vi "Aquitaine Editor.vi"(10 "Project Info":T5, 11 "Path":path) -> ()   [LabVIEW 2025]
uses:
  Types/Decision Tree.ctl
  Types/Sequencing Tree Node.ctl
  Types/Single Cmd Info.ctl
  <vilib>/picture/picture.llb/imagedata.ctl
  <vilib>/Utility/miscctls.llb/LVPositionTypeDef.ctl
panel:
  in  "Test Tree":T1
  out "AQT PATH NAME":string
  in  "Refresh":bool
  in  "Export to Draw Menu":bool
  in  "Close":bool
  out "Tree":picture
  out "Sequencing Command Palette":picture
  in  "Save":bool
  in  "Path References":i32[](listbox)
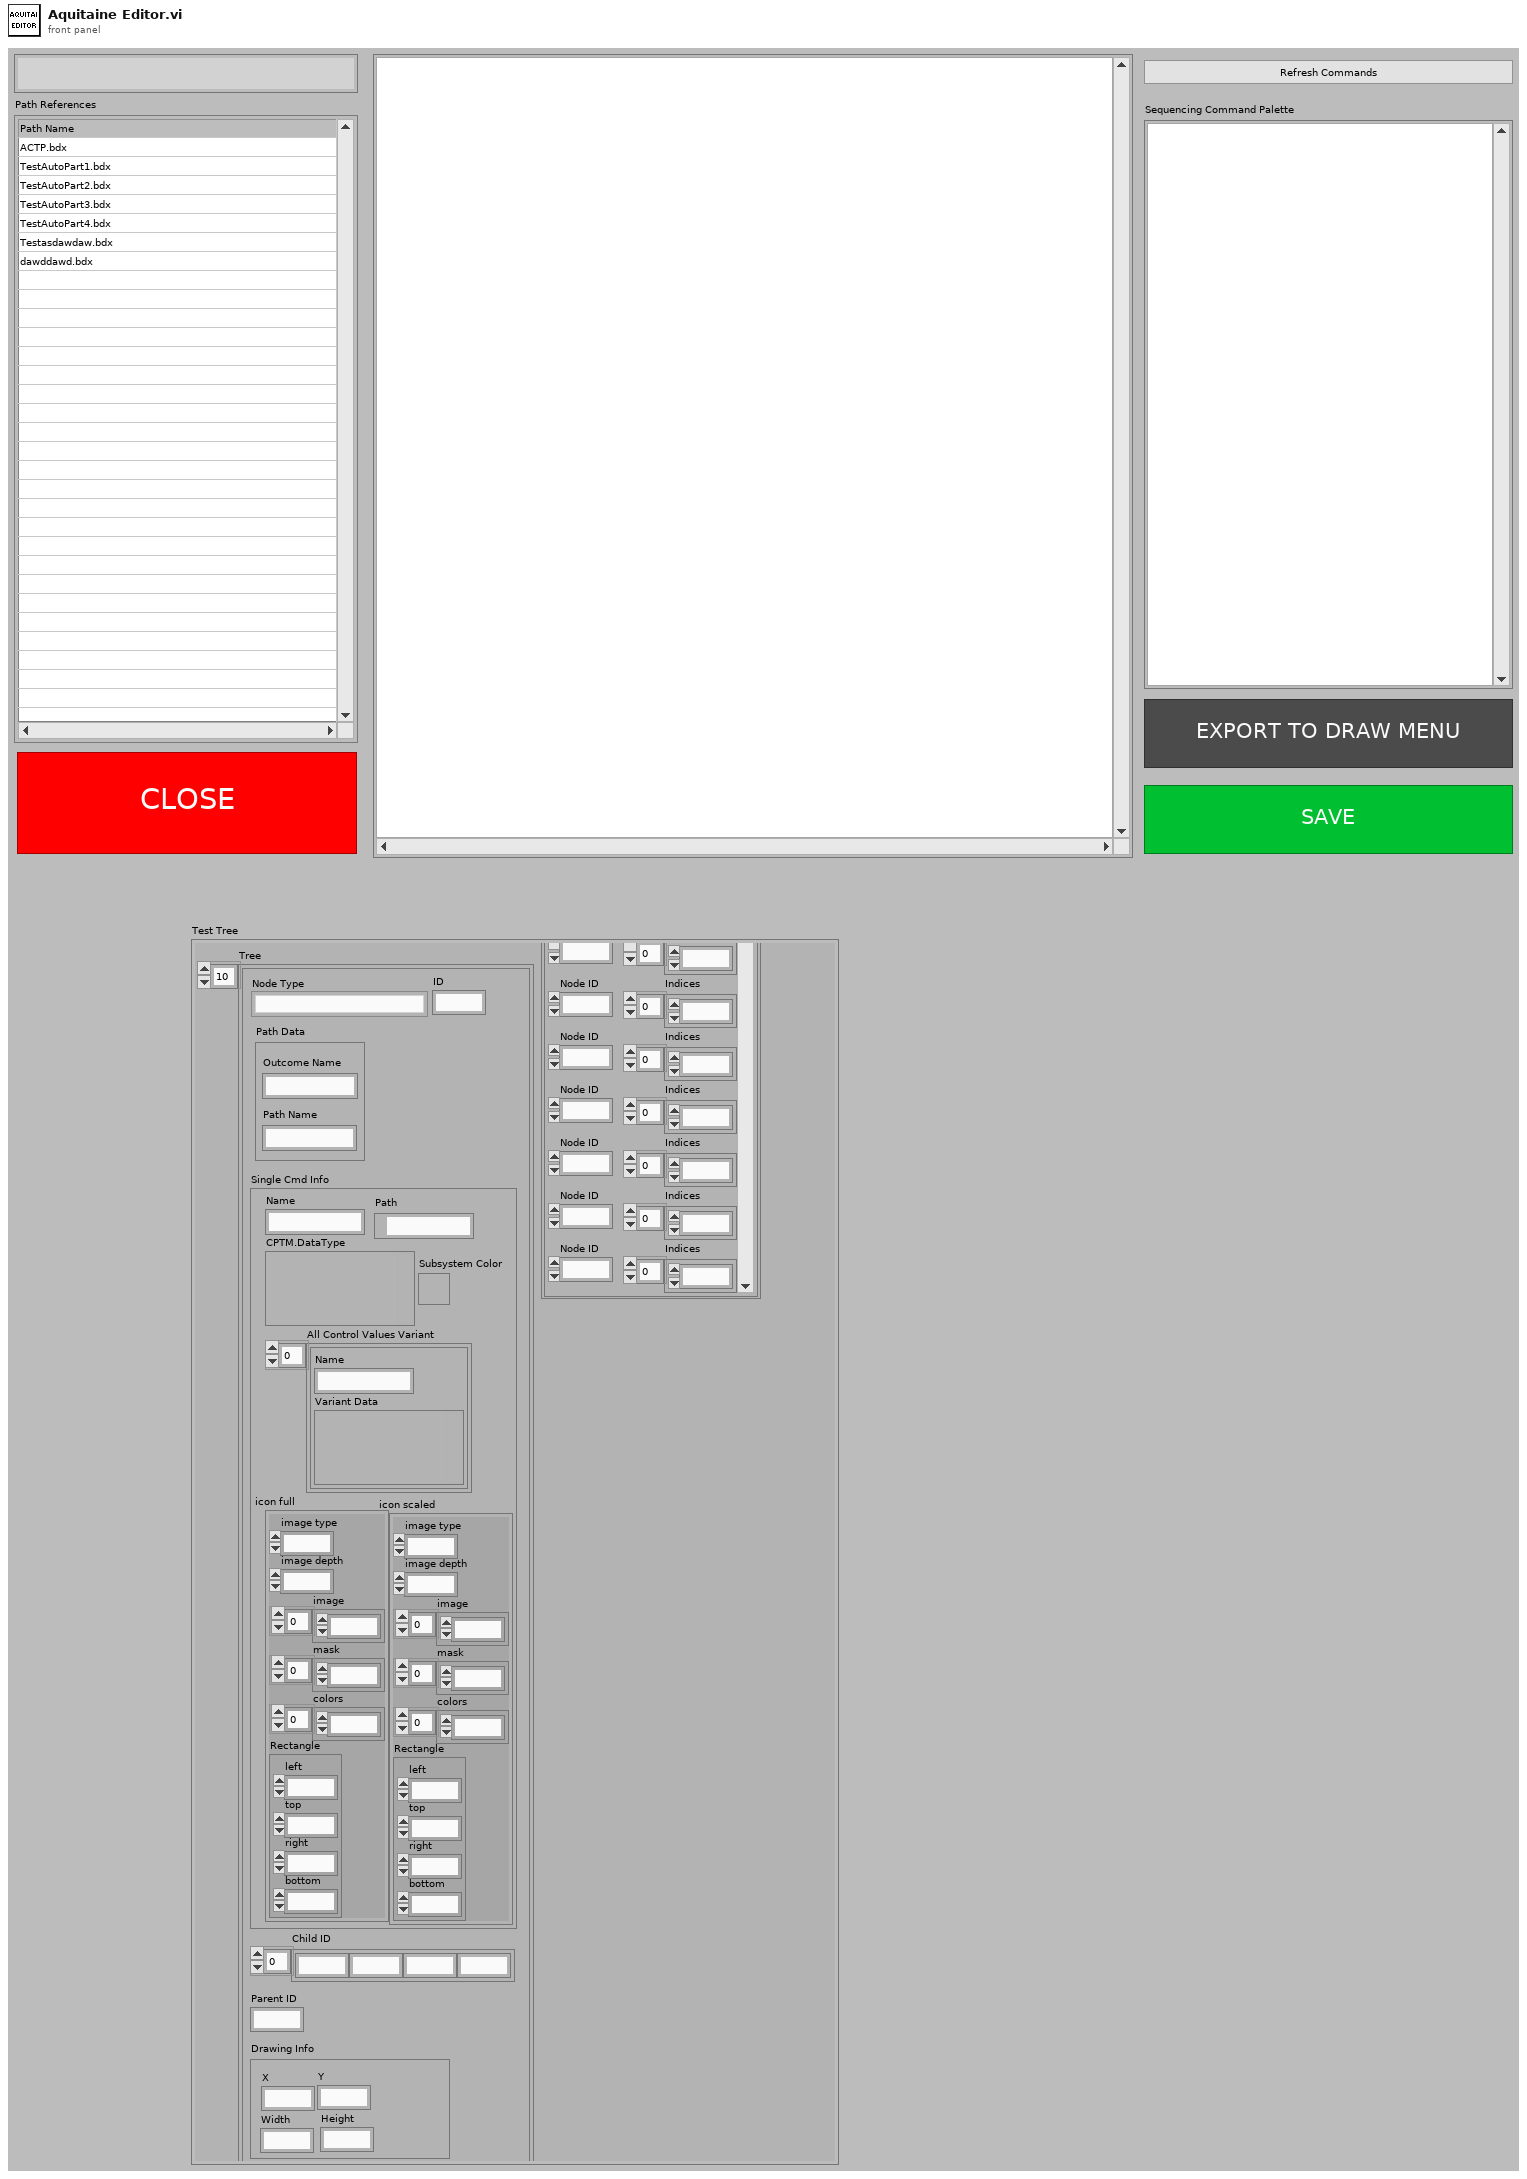
[diagram p1: front panel]
types:
  T1 = typedef "Decision Tree.ctl" = cluster{"Tree":T2[], "Node To Index Lookup Map":map{i16, i16[]}}
  T2 = typedef "Sequencing Tree Node.ctl" = cluster{"Node Type":enum16{"Path", "Command", "Leaf"}, "ID":i16, "Path Data":cluster{"Path Name":string, "Outcome Name":string}, "Single Cmd Info":T3, "Child ID":i32[], "Parent ID":i32, "Drawing Info":cluster{"X":i32, "Y":i32, "Width":i32, "Height":i32}}
  T3 = typedef "Single Cmd Info.ctl" = cluster{"Name":string, "CPTM.DataType":variant, "All Control Values Variant":cluster{"Name":string, "Variant Data":variant}[], "icon full":T4, "icon scaled":T4, "Path":path, "Subsystem Color":u32}
  T4 = typedef "imagedata.ctl" = cluster{"image type":i32, "image depth":i32, "image":u8[], "mask":u8[], "colors":u32[], "Rectangle":cluster{"left":i16, "top":i16, "right":i16, "bottom":i16}}
  T5 = cluster{"Targets":refnum<vi>[], "Paths":path[], "Projects":u16}
  T6 = typedef "LVPositionTypeDef.ctl" = cluster{"Left":i32, "Top":i32}
  T7 = cluster{"Path References":path[], "Decision Tree":T1}
  T8 = typedef "LVBoundsTypeDef.ctl" = cluster{"Width":u32, "Height":u32}
  T9 = cluster{"Shift":bool, "Ctrl":bool, "Alt":bool, "Cmd":bool, "Opt":bool}
  T10 = typedef "LVMouseTypeDef.ctl" = cluster{"Mouse Position":cluster{"X":i32, "Y":i32}, "Mouse Modifiers":cluster{"Button Down":bool, "Shift Mod":bool, "Menu Mod":bool, "Option Mod":bool}}
  T11 = cluster{"Tree Out":T2[], "map out":map{i16, i16[]}}
  T12 = typedef "eventvkey.ctl" = enum16{"ASCII", "Enter", "Return", "Shift", "Ctrl", "Alt", "Cmd", "Opt", "Caps", "NumLock", "Clear", "Break", "Up", "Down", "Left", "Right", "Insert", "Delete", "Home", "End", "PageUp", "PageDown", "Escape", "Help", "Pause", "ScrollLock", "F1", "F2", "F3", "F4", "F5", "F6", "F7", "F8", "F9", "F10", "F11", "F12", "F13", "F14", "F15", "F16", "F17", "F18", "F19", "F20", "F21", "F22", "F23", "F24", "Play", "VolumeUp", "VolumeDown", "Mute", "Two Byte Char"}
  T13 = typedef "LVPoint32TypeDef.ctl" = cluster{"Horizontal":i32, "Vertical":i32}
  T14 = typedef "LVRowAndColumnTypeDef.ctl" = cluster{"Row":i32, "Column":i32}
  T15 = cluster{"Tree":T2[], "Node To Index Lookup Map":map{i16, i16[]}}
  T16 = cluster{"Name":string, "CPTM.DataType":variant, "Get All Control Values Variant":cluster{"Name":string, "Variant Data":variant}[], "Color 256":T4, "Subsystem Color":u32}[]
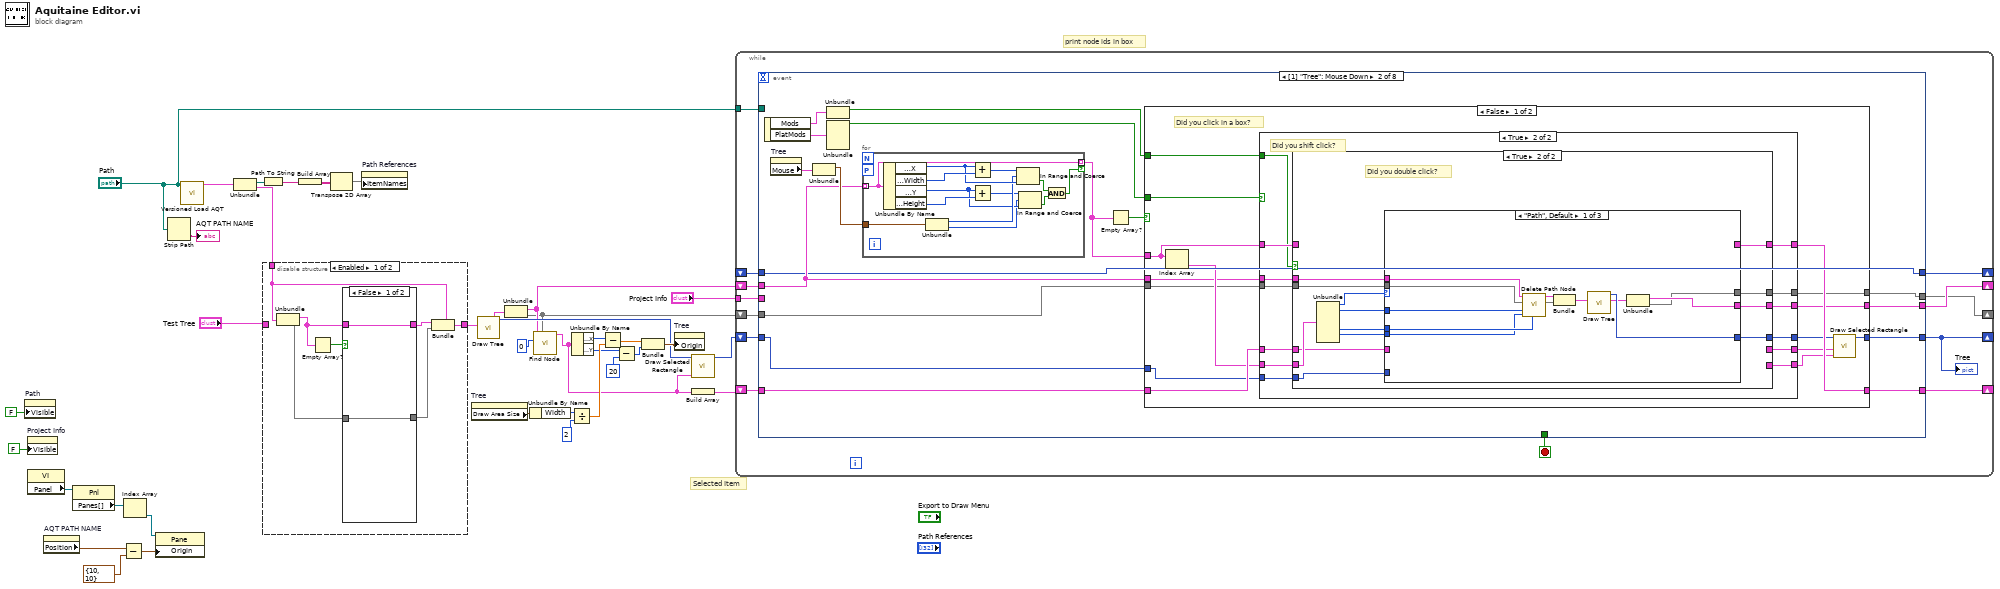
[diagram p0: block diagram]
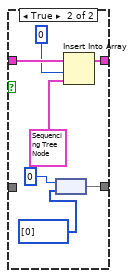
[diagram p2: hidden frame]
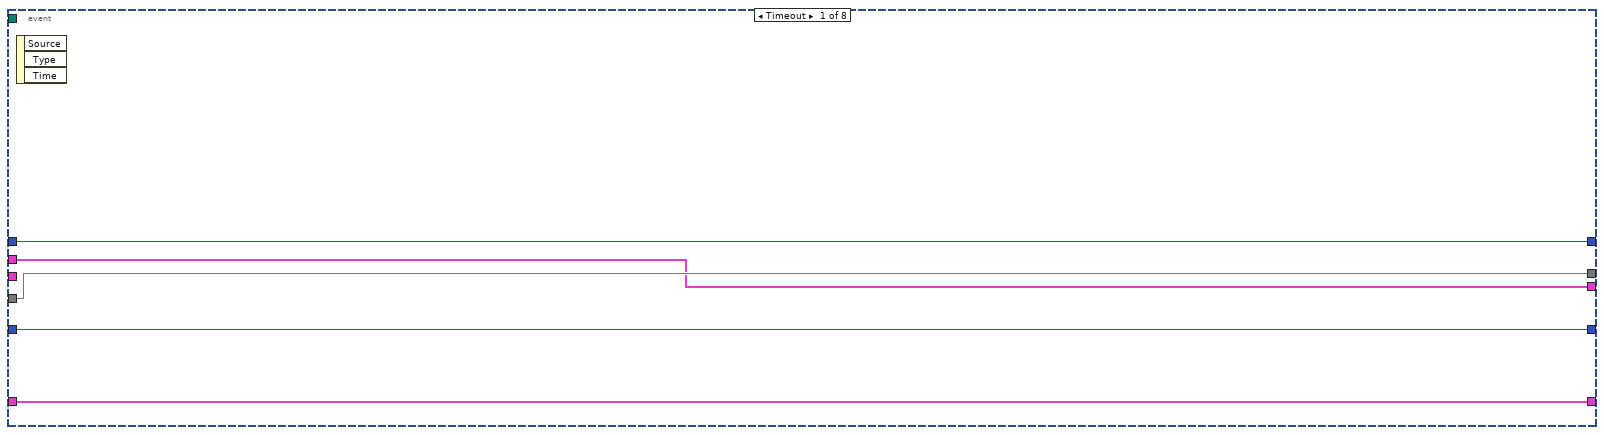
[diagram p4: hidden frame]
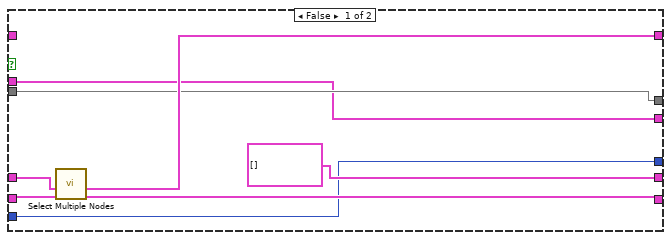
[diagram p6: hidden frame]
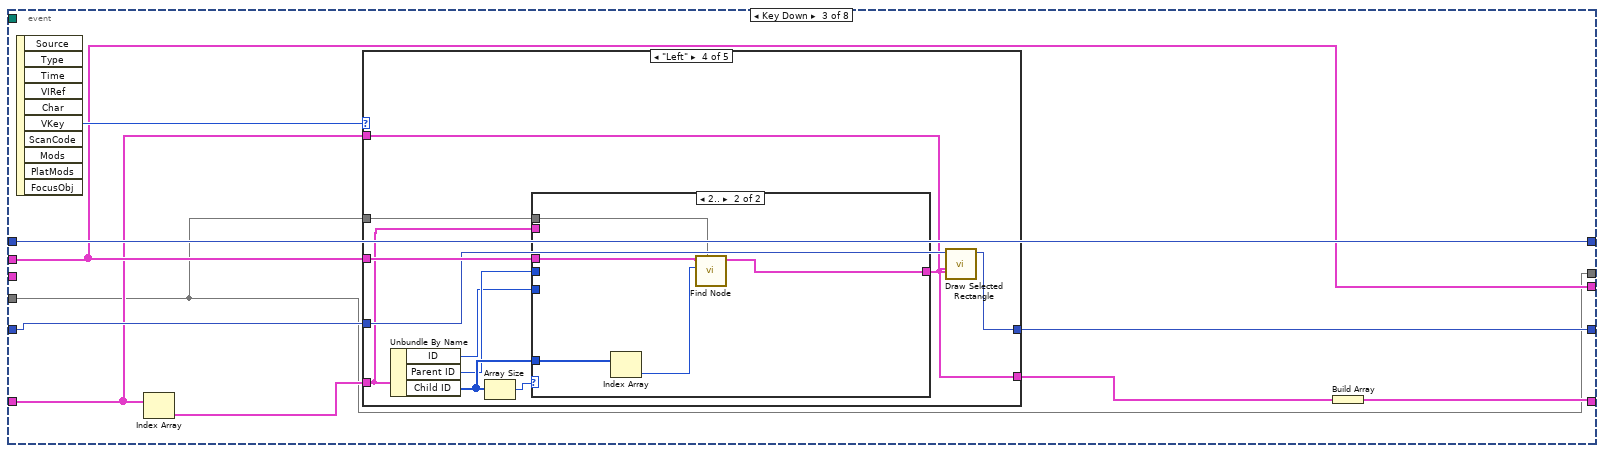
[diagram p10: hidden frame]
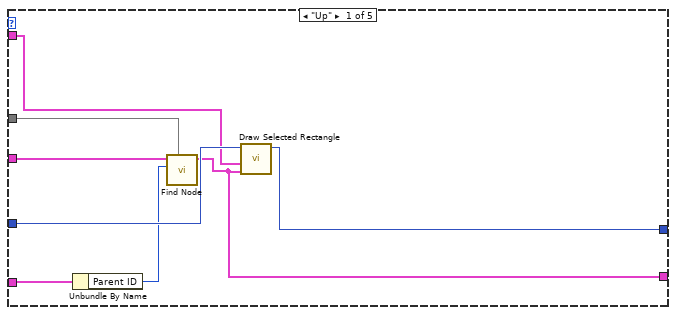
[diagram p11: hidden frame]
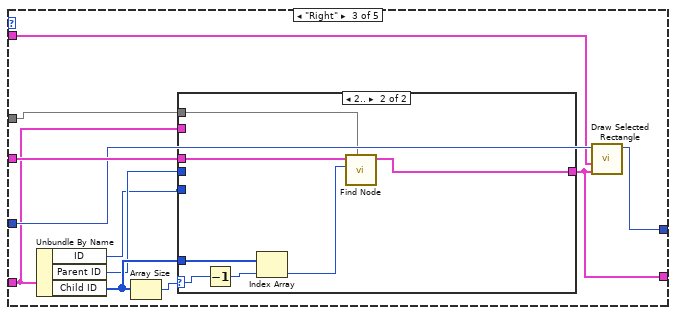
[diagram p13: hidden frame]
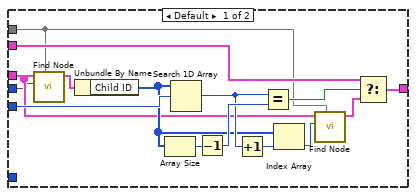
[diagram p14: hidden frame]
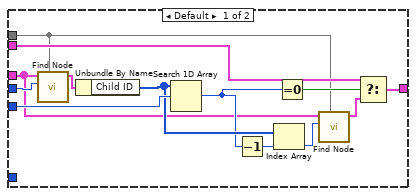
[diagram p15: hidden frame]
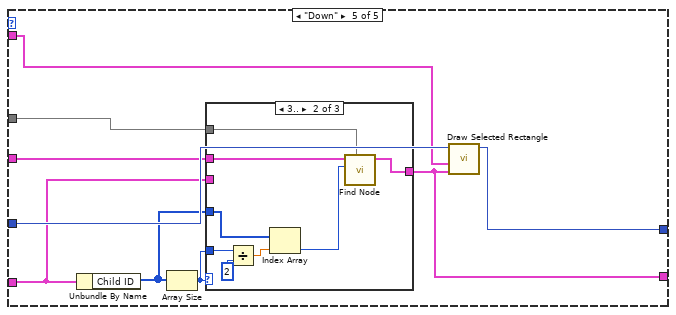
[diagram p16: hidden frame]
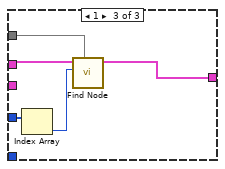
[diagram p18: hidden frame]
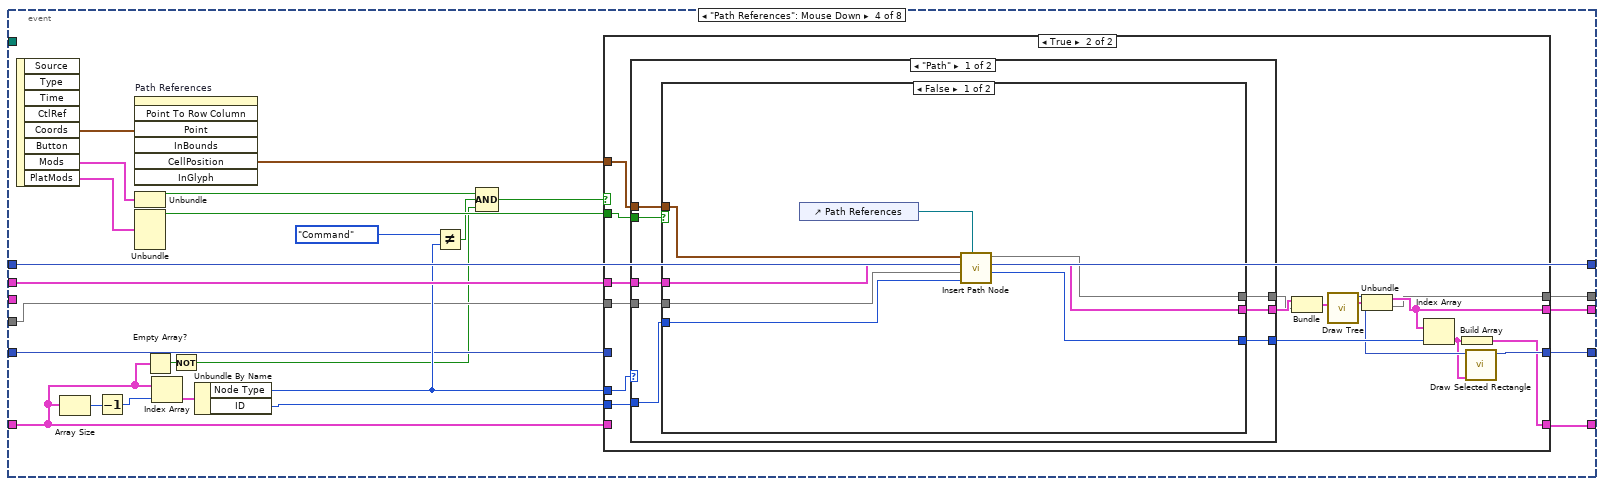
[diagram p19: hidden frame]
diagram:
  # "print node ids in box"
  # "Selected Item"
  n1 = property on="Path" class="Path"("Visible"=FALSE) -> ()  [unwired: 2 in, 2 out]
  n2 = property on="Project Info" class="Clust (strict)"("Visible"=FALSE) -> ()  [unwired: 2 in, 2 out]
  n3 = property class="VI"() -> ("Panel"=w27:refnum<vi>)  [unwired: 2 in, 2 out]
  n4 = property on="AQT PATH NAME" class="Str"() -> ("Position"=w23:T6)  [unwired: 2 in, 2 out]
  n5 = property class="Pnl"(reference=w27) -> ("Panes[]"=w26:refnum<vi>[])  [unwired: 1 in, 2 out]
  n6 = Subtract(x=w23, y=T6 {"Left"=10, "Top"=10}) -> (x-y=w22:T6)
  n7 = Index Array(array=w26) -> (element=w25:refnum<vi>)  [unwired: 1 in]
  n8 = property class="Pane"(reference=w25, "Origin"=w22) -> ()  [unwired: 1 in, 2 out]
  n9 = Strip Path(path="Path") -> (name=→"AQT PATH NAME":string)  [unwired: 1 out]
  n10 = call "Versioned Load AQT.vi"("Path"="Path") -> ("data"=w37:T7)  [unwired: 10 in]
  n11 = Unbundle(w37) -> ("Path References"=w36:path[], "Decision Tree"=w21:T1)
  n12 = Path To String(path=w36) -> (string=w35:string[])
  n13 = disable-structure shown="Enabled" {
    disable-tunnel: w21 -> [w41 _]
    disable-tunnel: [w40 w54] -> w8
    disable-tunnel: "Test Tree" -> [_ w54]
    frame Enabled {
      n14 = Unbundle(w41) -> ("Tree"=w43:T2[], "Node To Index Lookup Map"=w39:map{i16, i16[]})
      n15 = Empty Array?(array=w43) -> (empty?=w44:bool)
      n16 = case shown="False" w44 {
        tunnel: w43 -> [w46 w53]
        tunnel: [w46 w50] -> w42
        tunnel: w39 -> [w45 _]
        tunnel: [w45 w49] -> w38
        frame False {
        }
        frame True {
          n17 = node(i16 0, i16[] [0]) -> (w49:map{i16, i16[]})
          n18 = Insert Into Array(array=w53, index=0, new element=T2 {"Node Type"=enum."Leaf", "ID"=0, "Path Data"={"Path Name"="", "Outcome Name"=""}, "Single Cmd Info"={"Name"="", "CPTM.DataType"=variant, "All Control Values Variant"=[], "icon full"={"image type"=0, "image depth"=0, "image"=[], "mask"=[], "colors"=[], "Rectangle"={"left"=0, "top"=0, "right"=0, "bottom"=0}}, "icon scaled"={"image type"=0, "image depth"=0, "image"=[], "mask"=[], "colors"=[], "Rectangle"={"left"=0, "top"=0, "right"=0, "bottom"=0}}, "Path"=path "", "Subsystem Color"=16777216}, "Child ID"=[], "Parent ID"=0, "Drawing Info"={"X"=0, "Y"=0, "Width"=0, "Height"=0}} ("new element/subarray")) -> (w50:T2[])
        }
      }
      n19 = Bundle(cluster=w41, "Tree"=w42, "Node To Index Lookup Map"=w38) -> (w40:T1)
    }
    frame Disabled {
    }
  }
  n20 = Build Array(w35) -> (w34:string[][])
  n21 = Transpose 2D Array(2D array=w34) -> (transposed array=w33:string[][])
  n22 = property on="Path References" class="MCListbox (strict)"("ItemNames"=w33) -> ()  [unwired: 2 in, 2 out]
  n23 = property on="Tree" class="Pict"() -> ("Draw Area Size"=w17:T8)  [unwired: 2 in, 2 out]
  n24 = call "Draw Tree.vi"("Sequencing Data"=w8) -> ("Tree"=w5:T1, "2D Picture"=w10:picture)  [unwired: 9 in]
  n25 = Unbundle(w5) -> ("Tree"=w2:T2[], "Node To Index Lookup Map"=w1:map{i16, i16[]})
  n26 = Unbundle By Name(w17) -> ("Width"=w16:u32)
  n27 = call "Find Node.vi"("Node To Index Lookup Map"=w1, "ID"=0, "Tree"=w2) -> ("Node"=w3:T2)  [unwired: 7 in, 1 out]
  n28 = Divide(x=w16, y=u32 2) -> (x/y=w14:dbl)
  n29 = Unbundle By Name(w3) -> ("Drawing Info.X"=w19:i32, "Drawing Info.Y"=w12:i32)
  n30 = Subtract(x=w19, y=w14) -> (x-y=w18:dbl)
  n31 = Subtract(x=w12, y=20) -> (x-y=w13:i32)
  n32 = Bundle(w18, w13) -> (w20:cluster{dbl, i32})  [unwired: 1 in]
  n33 = property on="Tree" class="Pict"("Origin"=w20) -> ()  [unwired: 2 in, 2 out]
  n34 = call "Draw Selected Rectangle.vi"("New Node"=w3, "2D Picture"=w10) -> ("Decision Tree Out"=w9:picture)  [unwired: 9 in]
  n35 = Build Array(w3) -> (w6:T2[])
  n36 = while {
    tunnel: "Path" -> [w67]
    tunnel: "Project Info" -> [w65]
    shift-right: [w64] -> _
    shift-left: _ -> [w63]
    shift-right: [w58] -> _
    shift-left: w9 -> [w62]
    shift-right: [w59] -> _
    shift-left: w6 -> [w61]
    shift-right: [w56] -> _
    shift-left: w2 -> [w60]
    shift-right: [w55] -> _
    shift-left: w1 -> [w57]
    stop <- w66 stop-if-true
    n37 = event shown="[1] \"Tree\": Mouse Down" {
      selector: _ -> [_ _ _ _ _ _ _ _]
      dyn-events: _ -> [_ _ _ _ _ _ _ _]
      timeout: _ -> [_ _ _ _ _ _ _ _]
      tunnel: w67 -> [_ _ _ _ _ _ _ _]
      tunnel: [_ _ _ _ w392 _ _ w450] -> w66
      tunnel: w65 -> [_ _ _ _ _ w399 _ _]
      tunnel: [w72 w73 w190 w310 w391 w398 w427 w449] -> w64
      tunnel: w63 -> [w72 w73 w190 w310 w391 w397 w427 w449]
      tunnel: [w71 w80 w186 w290 w390 w396 w426 w448] -> w58
      tunnel: w62 -> [w71 w81 w188 w289 w390 w396 w426 w448]
      tunnel: w61 -> [w70 w84 w182 w288 w389 w395 w425 w447]
      tunnel: w60 -> [w68 w78 w187 w306 w387 w393 w423 w445]
      tunnel: [w70 w83 w183 w291 w389 w395 w425 w447] -> w59
      tunnel: w57 -> [w69 w77 w181 w294 w388 w394 w424 w446]
      tunnel: [w68 w75 w187 w293 w387 w393 w423 w445] -> w56
      tunnel: [w69 w74 w181 w292 w388 w394 w424 w446] -> w55
      event Timeout {
        n38 = event-data() -> ()  [unwired: 1 in, 3 out]
      }
      event "Tree": Mouse Down {
        n39 = event-data() -> ("Mods"=w88:cluster{"Double Click":bool, "Menu Key":bool}, "PlatMods"=w87:T9)  [unwired: 1 in]
        n40 = property on="Tree" class="Pict"() -> ("Mouse"=w89:T10)  [unwired: 2 in, 2 out]
        n41 = Unbundle(w89) -> ("Mouse Position"=w86:cluster{"X":i32, "Y":i32})  [unwired: 1 out]
        n42 = Unbundle(w88) -> ("Double Click"=w76:bool)  [unwired: 1 out]
        n43 = Unbundle(w87) -> ("Shift"=w79:bool)  [unwired: 4 out]
        n44 = for {
          workers-P: _ -> [_]
          tunnel: w78 -> [w91] mode=indexing
          tunnel: w86 -> [w102]
          tunnel: [w91] -> w82 mode=indexing if=w90
          n45 = Unbundle By Name(w91) -> ("Drawing Info.X"=w99:i32, "Drawing Info.Width"=w101:i32, "Drawing Info.Y"=w95:i32, "Drawing Info.Height"=w97:i32)
          n46 = Unbundle(w102) -> ("X"=w98:i32, "Y"=w94:i32)
          n47 = Add(x=w99, y=w101) -> (x+y=w100:i32)
          n48 = Add(x=w95, y=w97) -> (x+y=w96:i32)
          n49 = In Range and Coerce(upper limit=w100, x=w98, lower limit=w99) -> (In Range?=w92:bool)  [unwired: 1 out]
          n50 = In Range and Coerce(upper limit=w96, x=w94, lower limit=w95) -> (In Range?=w93:bool)  [unwired: 1 out]
          n51 = And(x=w92, y=w93) -> (x .and. y?=w90:bool)
        }
        n52 = Empty Array?(array=w82) -> (empty?=w85:bool)
        n53 = case shown="False" w85 {
          tunnel: w84 -> [w114 w180]
          tunnel: [w115 w180] -> w83
          tunnel: w82 -> [w116 _]
          tunnel: w81 -> [w104 w179]
          tunnel: [w117 w179] -> w80
          tunnel: w79 -> [w110 _]
          tunnel: w78 -> [w109 w177]
          tunnel: w77 -> [w108 w178]
          tunnel: w76 -> [w107 _]
          tunnel: [w106 w177] -> w75
          tunnel: [w105 w178] -> w74
          frame False {
            # "Did you click in a box?"
            n54 = Index Array(array=w116) -> (element=w112:T2)  [unwired: 1 in]
            n55 = case shown="True" w110 {
              tunnel: w116 -> [w123 w135]
              tunnel: [w123 w131] -> w115
              tunnel: w114 -> [w122 w132]
              tunnel: [w122 w136] -> w113
              tunnel: w112 -> [w121 w134]
              tunnel: [w121 w133] -> w111
              tunnel: w109 -> [w119 w130]
              tunnel: w108 -> [w120 w129]
              tunnel: w107 -> [_ w128]
              tunnel: [w119 w127] -> w106
              tunnel: [w120 w126] -> w105
              tunnel: w104 -> [w118 w125]
              tunnel: [w118 w124] -> w103
              frame False {
              }
              frame True {
                # "Did you shift click?"
                n56 = case shown="True" w128 {
                  tunnel: [T2[] [] ("Array") _] -> w136
                  tunnel: [w141 _] -> w133
                  tunnel: w135 -> [_ _]
                  tunnel: w134 -> [w142 w157]
                  tunnel: w132 -> [w143 w153]
                  tunnel: [w140 w152] -> w131
                  tunnel: w130 -> [w138 w155]
                  tunnel: w129 -> [w139 w154]
                  tunnel: [w138 w148] -> w127
                  tunnel: [w139 w147] -> w126
                  tunnel: w125 -> [w137 w146]
                  tunnel: [w137 w145] -> w124
                  frame False {
                    n57 = call "Select Multiple Nodes.vi"("Node to Select"=w142, "Selected Nodes"=w143) -> ("New Node"=w141:T2, "Selected Nodes New"=w140:T2[])  [unwired: 8 in]
                  }
                  frame True {
                    # "Did you double click?"
                    n58 = Unbundle(w157) -> ("Node Type"=w156:enum16{"Path", "Command", "Leaf"}, "ID"=w149:i16, "Child ID"=w150:i32[], "Parent ID"=w151:i32)  [unwired: 3 out]
                    n59 = case shown="\"Path\", Default" w156 {
                      tunnel: w155 -> [w168 w171 w175]
                      tunnel: w154 -> [w167 w172 w176]
                      tunnel: w153 -> [_ w173 _]
                      tunnel: [_ w173 _] -> w152
                      tunnel: w151 -> [w165 _ _]
                      tunnel: w150 -> [w169 _ _]
                      tunnel: w149 -> [w166 _ _]
                      tunnel: [w159 w171 w175] -> w148
                      tunnel: [w158 w172 w176] -> w147
                      tunnel: w146 -> [_ w170 w174]
                      tunnel: [w161 w170 w174] -> w145
                      frame "Path", Default {
                        n60 = call "Delete Path Node.vi"("Child ID"=w169, "Parent ID"=w165, "ID"=w166, "Node To Index Lookup Map"=w167, "Tree"=w168) -> ("map out"=w163:map{i16, i16[]}, "Tree Out"=w164:T2[])  [unwired: 5 in]
                        n61 = Bundle("Tree Out"=w164, "map out"=w163) -> (w162:T11)  [unwired: 1 in]
                        n62 = call "Draw Tree.vi"("Sequencing Data"=w162) -> ("Tree"=w160:T1, "2D Picture"=w161:picture)  [unwired: 9 in]
                        n63 = Unbundle(w160) -> ("Tree"=w159:T2[], "Node To Index Lookup Map"=w158:map{i16, i16[]})
                      }
                      frame "Leaf" {
                      }
                      frame "Command" {
                      }
                    }
                  }
                }
              }
            }
            n64 = call "Draw Selected Rectangle.vi"("New Node"=w111, "Prev. Node"=w113, "2D Picture"=w103) -> ("Decision Tree Out"=w117:picture)  [unwired: 8 in]
          }
          frame True {
          }
        }
      }
      event Key Down {
        n65 = event-data() -> ("VKey"=w189:T12)  [unwired: 1 in, 9 out]
        n66 = Index Array(array=w182) -> (element=w185:T2)  [unwired: 1 in]
        n67 = case shown="\"Left\"" w189 {
          tunnel: w188 -> [w198 w200 w208 w241 w271]
          tunnel: w185 -> [w196 w199 w205 w237 w265]
          tunnel: w187 -> [w194 _ w209 w242 w268]
          tunnel: [w197 w200 w207 w240 w270] -> w186
          tunnel: [w192 w199 w206 w238 w266] -> w184
          tunnel: w182 -> [w195 _ w202 w235 w264]
          tunnel: w181 -> [w191 _ w201 w234 w263]
          frame "Up" {
            n68 = Unbundle By Name(w196) -> ("Parent ID"=w193:i32)
            n69 = call "Find Node.vi"("Node To Index Lookup Map"=w191, "ID"=w193, "Tree"=w194) -> ("Node"=w192:T2)  [unwired: 7 in, 1 out]
            n70 = call "Draw Selected Rectangle.vi"("New Node"=w192, "Prev. Node"=w195, "2D Picture"=w198) -> ("Decision Tree Out"=w197:picture)  [unwired: 8 in]
          }
          frame Default {
          }
          frame "Right" {
            n71 = Unbundle By Name(w205) -> ("ID"=w203:i16, "Parent ID"=w204:i32, "Child ID"=w210:i32[])
            n72 = Array Size(array=w210) -> (size(s)=w211:i32)
            n73 = case shown="2.." w211 {
              selector: w211 -> [_ w232]
              tunnel: w210 -> [_ w233]
              tunnel: w209 -> [w215 w230]
              tunnel: [w222 w228] -> w206
              tunnel: w204 -> [w214 _]
              tunnel: w203 -> [w226 _]
              tunnel: w205 -> [w223 _]
              tunnel: w201 -> [w212 w227]
              frame Default {
                n74 = call "Find Node.vi"("Node To Index Lookup Map"=w212, "ID"=w214, "Tree"=w215) -> ("Node"=w213:T2)  [unwired: 7 in, 1 out]
                n75 = Unbundle By Name(w213) -> ("Child ID"=w218:i32[])
                n76 = Array Size(array=w218) -> (size(s)=w219:i32)
                n77 = Search 1D Array(1D array=w218, element=w226) -> (index of element=w220:i32)  [unwired: 1 in]
                n78 = Decrement(x=w219) -> (x-1=w224:i32)
                n79 = Increment(x=w220) -> (x+1=w221:i32)
                n80 = Equal?(x=w220, y=w224) -> (x = y?=w225:bool)
                n81 = Index Array(array=w218, index=w221) -> (element=w217:i32)
                n82 = call "Find Node.vi"("Node To Index Lookup Map"=w212, "ID"=w217, "Tree"=w215) -> ("Node"=w216:T2)  [unwired: 7 in, 1 out]
                n83 = Select(t=w223, s=w225, f=w216) -> (s? t:f=w222:T2)
              }
              frame 2.. {
                n84 = Decrement(x=w232) -> (x-1=w231:i32)
                n85 = Index Array(array=w233, index=w231) -> (element=w229:i32)
                n86 = call "Find Node.vi"("Node To Index Lookup Map"=w227, "ID"=w229, "Tree"=w230) -> ("Node"=w228:T2)  [unwired: 7 in, 1 out]
              }
            }
            n87 = call "Draw Selected Rectangle.vi"("New Node"=w206, "Prev. Node"=w202, "2D Picture"=w208) -> ("Decision Tree Out"=w207:picture)  [unwired: 8 in]
          }
          frame "Left" {
            n88 = Unbundle By Name(w237) -> ("ID"=w236:i16, "Parent ID"=w239:i32, "Child ID"=w243:i32[])
            n89 = Array Size(array=w243) -> (size(s)=w244:i32)
            n90 = case shown="2.." w244 {
              tunnel: w243 -> [_ w262]
              tunnel: w242 -> [w248 w261]
              tunnel: [w254 w259] -> w238
              tunnel: w239 -> [w250 _]
              tunnel: w236 -> [w257 _]
              tunnel: w237 -> [w255 _]
              tunnel: w234 -> [w245 w258]
              frame Default {
                n91 = call "Find Node.vi"("Node To Index Lookup Map"=w245, "ID"=w250, "Tree"=w248) -> ("Node"=w249:T2)  [unwired: 7 in, 1 out]
                n92 = Unbundle By Name(w249) -> ("Child ID"=w252:i32[])
                n93 = Search 1D Array(1D array=w252, element=w257) -> (index of element=w251:i32)  [unwired: 1 in]
                n94 = Decrement(x=w251) -> (x-1=w253:i32)
                n95 = Index Array(array=w252, index=w253) -> (element=w247:i32)
                n96 = Equal To 0?(x=w251) -> (x = 0?=w256:bool)
                n97 = call "Find Node.vi"("Node To Index Lookup Map"=w245, "ID"=w247, "Tree"=w248) -> ("Node"=w246:T2)  [unwired: 7 in, 1 out]
                n98 = Select(t=w255, s=w256, f=w246) -> (s? t:f=w254:T2)
              }
              frame 2.. {
                n99 = Index Array(array=w262) -> (element=w260:i32)  [unwired: 1 in]
                n100 = call "Find Node.vi"("Node To Index Lookup Map"=w258, "ID"=w260, "Tree"=w261) -> ("Node"=w259:T2)  [unwired: 7 in, 1 out]
              }
            }
            n101 = call "Draw Selected Rectangle.vi"("New Node"=w238, "Prev. Node"=w235, "2D Picture"=w241) -> ("Decision Tree Out"=w240:picture)  [unwired: 8 in]
          }
          frame "Down" {
            n102 = Unbundle By Name(w265) -> ("Child ID"=w269:i32[])
            n103 = Array Size(array=w269) -> (size(s)=w267:i32)
            n104 = case shown="3.." w267 {
              tunnel: w269 -> [_ w277 w285]
              tunnel: w268 -> [_ w276 w283]
              tunnel: [w272 w273 w281] -> w266
              tunnel: w265 -> [w272 _ _]
              tunnel: w267 -> [_ w280 _]
              tunnel: w263 -> [_ w274 w282]
              frame 0, Default {
              }
              frame 3.. {
                n105 = Divide(x=w280, y=2) -> (x/y=w278:dbl)
                n106 = Index Array(array=w277, index=w278) -> (element=w275:i32)
                n107 = call "Find Node.vi"("Node To Index Lookup Map"=w274, "ID"=w275, "Tree"=w276) -> ("Node"=w273:T2)  [unwired: 7 in, 1 out]
              }
              frame 1 {
                n108 = Index Array(array=w285) -> (element=w284:i32)  [unwired: 1 in]
                n109 = call "Find Node.vi"("Node To Index Lookup Map"=w282, "ID"=w284, "Tree"=w283) -> ("Node"=w281:T2)  [unwired: 7 in, 1 out]
              }
            }
            n110 = call "Draw Selected Rectangle.vi"("New Node"=w266, "Prev. Node"=w264, "2D Picture"=w271) -> ("Decision Tree Out"=w270:picture)  [unwired: 8 in]
          }
        }
        n111 = Build Array(w184) -> (w183:T2[])
      }
      event "Path References": Mouse Down {
        n112 = event-data() -> ("Coords"=w309:T13, "Mods"=w308:cluster{"Double Click":bool, "Menu Key":bool}, "PlatMods"=w307:T9)  [unwired: 1 in, 5 out]
        n113 = Array Size(array=w288) -> (size(s)=w303:i32)
        n114 = Decrement(x=w303) -> (x-1=w302:i32)
        n115 = invoke on="Path References" class="MCListbox (strict)" method="Point To Row Column"("Point"=w309) -> ("CellPosition"=w305:T14)  [unwired: 6 in, 6 out]
        n116 = Unbundle(w308) -> ("Double Click"=w299:bool)  [unwired: 1 out]
        n117 = Unbundle(w307) -> ("Shift"=w304:bool)  [unwired: 4 out]
        n118 = Empty Array?(array=w288) -> (empty?=w287:bool)
        n119 = Index Array(array=w288, index=w302) -> (element=w301:T2)
        n120 = Not(x=w287) -> (.not. x?=w286:bool)
        n121 = Unbundle By Name(w301) -> ("Node Type"=w296:enum16{"Path", "Command", "Leaf"}, "ID"=w295:i16)
        n122 = Not Equal?(x=enum16{"Path", "Command", "Leaf"}."Command", y=w296) -> (x != y?=w298:bool)
        n123 = Compound Arithmetic op=AND(w299, w298, w286) -> (w300:bool)
        n124 = case shown="True" w300 {
          tunnel: w306 -> [w314 w331]
          tunnel: w305 -> [_ w327]
          tunnel: w304 -> [_ w315]
          tunnel: w296 -> [_ w330]
          tunnel: w295 -> [_ w329]
          tunnel: w294 -> [w313 w328]
          tunnel: [w314 w326] -> w293
          tunnel: [w313 w325] -> w292
          tunnel: [w312 w323] -> w291
          tunnel: w288 -> [w312 _]
          tunnel: [w311 w324] -> w290
          tunnel: w289 -> [w311 _]
          frame False {
          }
          frame True {
            n125 = case shown="\"Path\"" w330 {
              tunnel: w329 -> [w339 w370]
              tunnel: w331 -> [w338 w366]
              tunnel: w328 -> [w335 w369]
              tunnel: w327 -> [w337 w383]
              tunnel: [w336 w373] -> w322
              tunnel: [w333 w368] -> w321
              tunnel: [w334 w362] -> w318
              tunnel: w315 -> [w332 _]
              frame "Path" {
                n126 = case shown="False" w332 {
                  tunnel: w339 -> [w340 w361]
                  tunnel: w338 -> [w342 w360]
                  tunnel: w337 -> [w343 w358]
                  tunnel: [w345 w351] -> w336
                  tunnel: w335 -> [w341 w348]
                  tunnel: [w346 w349] -> w334
                  tunnel: [w347 w348] -> w333
                  frame False {
                    n127 = control-ref of="Path References"() -> (w344:refnum<vi>)
                    n128 = call "Insert Path Node.vi"("MulticolumnListbox in"=w344, "ID"=w340, "Node To Index Lookup Map in"=w341, "Tree"=w342, "CellPosition"=w343) -> ("Index of Selected Node"=w346:i32, "Tree Out"=w345:T2[], "Node To Index Lookup Map out"=w347:map{i16, i16[]})  [unwired: 4 in]
                  }
                  frame True {
                    # "Replace the item with the path"
                    n129 = call "Find Node.vi"("Node To Index Lookup Map"=w348, "ID"=w361, "Tree"=w360) -> ("Index"=w349:i16, "Node"=w354:T2)  [unwired: 7 in]
                    n130 = property on="Path References" class="MCListbox (strict)"() -> ("ItemNames"=w359:string[][])  [unwired: 2 in, 2 out]
                    n131 = Unbundle(w358) -> ("Row"=w357:i32, "Column"=w356:i32)
                    n132 = Unbundle By Name(w354) -> ("Path Data.Outcome Name"=w353:string)
                    n133 = Index Array(array=w359, index (row)=w357, index (col)=w356) -> (element=w355:string)
                    n134 = Bundle(w355, "Outcome Name"=w353) -> (w352:cluster{string, "Outcome Name":string})  [unwired: 1 in]
                    n135 = Bundle(cluster=w354, "Path Data"=w352) -> (w350:T2)  [unwired: 6 in]
                    n136 = Replace Array Subset(array=w360, new element=w350, index=w349) -> (w351:T2[])
                  }
                }
              }
              frame "Leaf", Default {
                n137 = call "Find Node.vi"("Node To Index Lookup Map"=w369, "ID"=w370, "Tree"=w366) -> ("Index"=w386:i16, "Node"=w379:T2)  [unwired: 7 in]
                n138 = property on="Path References" class="MCListbox (strict)"() -> ("ItemNames"=w384:string[][])  [unwired: 2 in, 2 out]
                n139 = Unbundle(w383) -> ("Row"=w382:i32, "Column"=w381:i32)
                n140 = Unbundle By Name(w379) -> ("Path Data.Outcome Name"=w378:string)
                n141 = Read Map Max & Min Keys(11:w369) -> (3:w376:i16)  [unwired: 1 out]
                n142 = Index Array(array=w384, index (row)=w382, index (col)=w381) -> (element=w380:string)
                n143 = Increment(x=w376) -> (x+1=w367:i16)
                n144 = Bundle(w380, "Outcome Name"=w378) -> (w377:cluster{string, "Outcome Name":string})  [unwired: 1 in]
                n145 = Build Array(w367) -> (w375:i16[])
                n146 = Bundle(cluster=w379, "Node Type"=enum16{"Path", "Command", "Leaf"}."Path", "Path Data"=w377, "Child ID"=w375) -> (w385:T2)  [unwired: 4 in]
                n147 = Replace Array Subset(array=w366, new element=w385, index=w386) -> (w364:T2[])
                n148 = Bundle(cluster=T2 {"Node Type"=enum."Path", "ID"=0, "Path Data"={"Path Name"="", "Outcome Name"=""}, "Single Cmd Info"={"Name"="", "CPTM.DataType"=variant, "All Control Values Variant"=[], "icon full"={"image type"=0, "image depth"=0, "image"=[], "mask"=[], "colors"=[], "Rectangle"={"left"=0, "top"=0, "right"=0, "bottom"=0}}, "icon scaled"={"image type"=0, "image depth"=0, "image"=[], "mask"=[], "colors"=[], "Rectangle"={"left"=0, "top"=0, "right"=0, "bottom"=0}}, "Path"=path "", "Subsystem Color"=0}, "Child ID"=[], "Parent ID"=0, "Drawing Info"={"X"=0, "Y"=0, "Width"=0, "Height"=0}} ("Cluster"), "Node Type"=enum16{"Path", "Command", "Leaf"}."Leaf", "ID"=w367, "Parent ID"=w370) -> (w363:T2)  [unwired: 4 in]
                n149 = Array Size(array=w364) -> (size(s)=w362:i32)
                n150 = Build Array(w362) -> (w365:i32[])
                n151 = Insert Into Map(map in=w369, key=w367, value=w365) -> (map out=w368:map{i16, i16[]})  [unwired: 2 out]
                n152 = Build Array (concatenate)(w364, w363) -> (w373:T2[])
              }
            }
            n153 = Bundle("Tree"=w322, "Node To Index Lookup Map"=w321) -> (w320:T15)  [unwired: 1 in]
            n154 = call "Draw Tree.vi"("Sequencing Data"=w320) -> ("Tree"=w319:T1, "2D Picture"=w317:picture)  [unwired: 9 in]
            n155 = Unbundle(w319) -> ("Tree"=w326:T2[], "Node To Index Lookup Map"=w325:map{i16, i16[]})
            n156 = Index Array(array=w326, index=w318) -> (element=w316:T2)
            n157 = Build Array(w316) -> (w323:T2[])
            n158 = call "Draw Selected Rectangle.vi"("New Node"=w316, "2D Picture"=w317) -> ("Decision Tree Out"=w324:picture)  [unwired: 9 in]
          }
        }
      }
      event "Save": Value Change {
        n159 = event-data() -> ("NewVal"=w392:bool)  [unwired: 1 in, 5 out]
      }
      event "Refresh": Value Change {
        n160 = event-data() -> ("NewVal"=w400:bool)  [unwired: 1 in, 5 out]
        n161 = case shown="True" w400 {
          tunnel: w399 -> [_ w407]
          tunnel: [w401 w402] -> w398
          tunnel: w397 -> [w401 _]
          frame False {
          }
          frame True {
            n162 = flat-sequence {
              tunnel: w407 -> [w409]
              tunnel: [w409] -> w406
              tunnel: [w408] -> w405
              tunnel: w406 -> [w417]
              tunnel: w405 -> [w411]
              tunnel: [w411] -> w404
              tunnel: [w410] -> w403
              tunnel: w404 -> [w422]
              tunnel: w403 -> [w421]
              tunnel: [w421] -> w402
              frame #0 {
                n163 = call <vilib>:"Set Busy.vi"() -> ("error out"=w408:errorcluster)  [unwired: 10 in, 1 out]
              }
              frame #1 {
                n164 = Unbundle(w417) -> ("Targets"=w420:refnum<vi>[], "Paths"=w419:path[], "Projects"=w412:u16)
                n165 = Index Array(array=w420, index=w412) -> (element=w416:refnum<vi>)
                n166 = Index Array(array=w419, index=w412) -> (element=w418:path)
                n167 = Strip Path(path=w418) -> (stripped path=w415:path)  [unwired: 1 out]
                n168 = call "Find Sequencing Command Names.vi"("project root path"=w415, "TargetItem in"=w416) -> ("Paths"=w413:path[], "Command Info"=w414:T16)  [unwired: 8 in]
                n169 = call "Format Seqencing Command Pallet.vi"("Paths"=w413, "Command Info"=w414) -> ("2D Picture"=w410:picture)  [unwired: 8 in, 1 out]
                "Sequencing Command Palette" <- w410
              }
              frame #2 {
                n170 = call <vilib>:"Unset Busy.vi"("error in (no error)"=w422) -> ()  [unwired: 10 in, 1 out]
              }
            }
          }
        }
      }
      event "Sequencing Command Palette": Mouse Move {
        w429 = 35 ("Row Height")
        n171 = event-data() -> ("Coords"=w428:T13)  [unwired: 1 in, 4 out]
        n172 = control-ref of="Sequencing Command Palette"() -> (w430:refnum<vi>)
        n173 = call "Picture Coord to Row.vi"("Row Height"=w429, "Coords"=w428, "Picture in"=w430) -> ("Row Index"=w431:i32, "Clicked in canvas"=w432:bool)  [unwired: 7 in]
        n174 = case shown="True" w432 {
          tunnel: w431 -> [_ w437]
          tunnel: w429 -> [_ w434]
          tunnel: w427 -> [_ w433]
          frame False {
          }
          frame True {
            n175 = Multiply(x=w437, y=w434) -> (x*y=w440:i32)
            n176 = Add(x=w440, y=w434) -> (x+y=w441:i32)
            n177 = Bundle(0, w440, 300, w441) -> (w442:cluster{i32, i32, i32, i32})  [unwired: 1 in]
            n178 = call <vilib>:"Draw Rectangle.vi"("rect"=w442, "fill?(F)"=TRUE, "color(black)"=u32 10539263) -> ("new picture"=w436:picture)  [unwired: 6 in]
            n179 = Concatenate Strings(w436, w433) -> (w435:picture)
            n180 = local write "Sequencing Command Palette"(w435) -> ()
          }
        }
      }
      event "Close": Value Change {
        n181 = event-data() -> ("NewVal"=w450:bool)  [unwired: 1 in, 5 out]
      }
    }
    "Tree" <- w58
  }
